vi "Read Parameters to process.vi"(8 "error in":errorcluster, 11 "RTResourceUtilitzation runtime in":refnum<class "RTResourceUtilitzation runtime.lvclass">) -> (0 "error out":errorcluster, 2 "Parameters to process":T1, 3 "RTResourceUtilitzation runtime out":refnum<class "RTResourceUtilitzation runtime.lvclass">)   [LabVIEW 2014, in "RTResourceUtilitzation runtime.lvclass"]
uses:
  RTResourceUtilitzation runtime.lvclass
  configuration/parameter data indices.ctl
  RTResourceUtilitzation runtime.lvclass/RTResourceUtilitzation runtime.ctl
  configuration/RTResourceUtilitzation configuration.lvclass
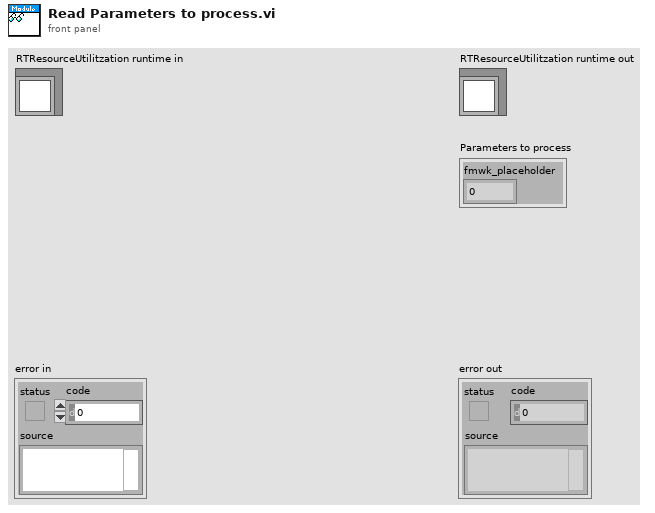
[diagram p1: front panel]
types:
  T1 = typedef "RTResourceUtilitzation configuration.lvclass/parameter data indices.ctl" = cluster{"fmwk_placeholder":i32}
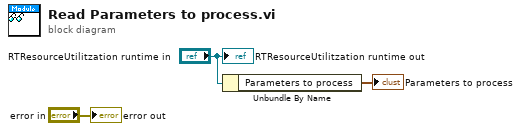
[diagram p0: block diagram]
diagram:
  n1 = Unbundle By Name("RTResourceUtilitzation runtime in") -> ("Parameters to process"=→"Parameters to process":T1)
  "error out" <- "error in"
  "RTResourceUtilitzation runtime out" <- "RTResourceUtilitzation runtime in"
